vi "Read H2 Sensor Values.vi"(8 "error in (no error)":errorcluster, 11 "Refnum in":refnum<k21>) -> (0 "error out":errorcluster, 1 "Data Map":map{string, dbl}(c390), 2 "data":dbl[](array[numeric]) format="%.2f", 3 "Refnum out":refnum<k21>)   [LabVIEW 2024, in "Anode.lvlib"]
uses:
  Anode.lvlib
  <vilib>/xnet/xnet.llb/XNET Read (Signal Single-point).vi
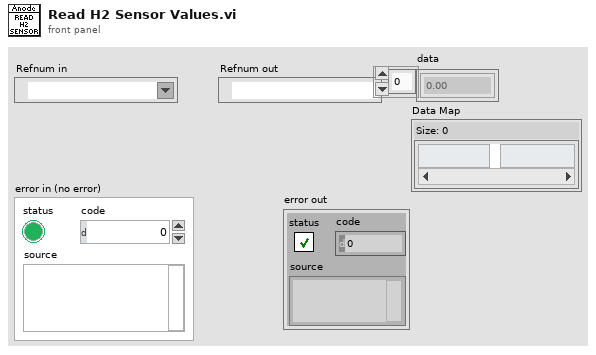
[diagram p1: front panel]
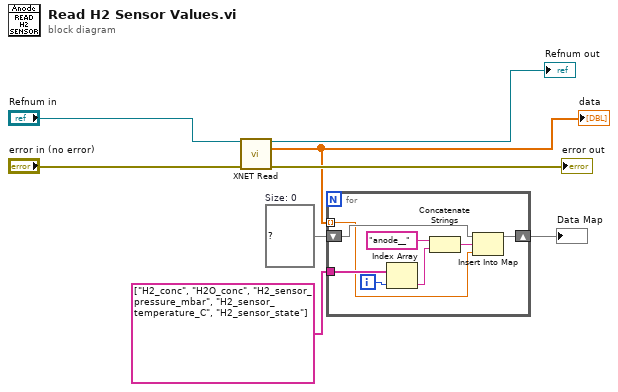
[diagram p0: block diagram]
diagram:
  w5 = map{string, dbl} {}  # Size: 0
  n1 = call-poly <vilib>:"XNET Read.vi"("session in"="Refnum in", "error in (no error)"="error in (no error)") -> ("session out"=→"Refnum out":refnum<k21>, "data"=w3:dbl[], "error out"=→"error out":errorcluster)  [unwired: 11 in]
  "data" <- w3
  n2 = for {
    tunnel: string[] ["H2_conc", "H2O_conc", "H2_sensor_pressure_mbar", "H2_sensor_temperature_C", "H2_sensor_state"] -> [w11]
    tunnel: w3 -> [w9] mode=indexing
    shift-right: [w16] -> w4
    shift-left: w5 -> [w15]
    i -> [w12]
    n3 = Index Array(array=w11, index=w12) -> (element=w10:string)
    n4 = Concatenate Strings("anode__", w10) -> (w13:string)
    n5 = Insert Into Map(map in=w15, key=w13, value=w9) -> (map out=w16:map{string, dbl})  [unwired: 2 out]
  }
  "Data Map" <- w4
